vi "ListaStringParametros.vi"(2 "Tipo":T1, 4 "Parametros":variant) -> (16 "Parametros":string[](array[string]))   [LabVIEW 2017]
uses:
  Typedefs/Tipo_TipoSinalSimulado.ctl
  Typedefs/Tipo_ParamsRuido.ctl
  Typedefs/Tipo_ParamsFasor.ctl
  Typedefs/Tipo_ParamsSenoide.ctl
  Typedefs/Tipo_ParamsComposto.ctl
  Typedefs/Tipo_ComponenteSinalComposto.ctl
  Typedefs/Tipo_ParamsAMgen.ctl
  Typedefs/Tipo_ComponenteSinalRuidoComposto.ctl
  Typedefs/Tipo_TipoSinalCarrier.ctl
  Typedefs/Tipo_ParamsProximeter.ctl
  Typedefs/Tipo_ComponentesProximeter.ctl
  Typedefs/Tipo_ParamsEntreferro.ctl
  Typedefs/Tipo_ComponenteSinalEntreferro.ctl
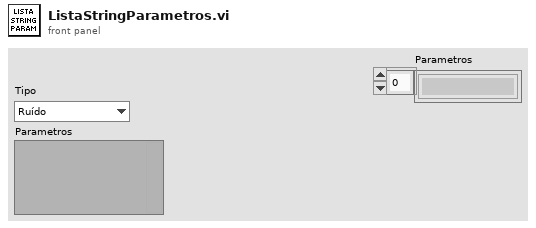
[diagram p1: front panel]
types:
  T1 = typedef "Tipo_TipoSinalSimulado.ctl" = enum16{"Ruído", "Fasor", "Senóide", "Composto", "AM", "Proximidade", "Entreferro"}
  T2 = typedef "Tipo_ParamsRuido.ctl" = cluster{"Amplitude":dbl, "Banda: ":bool, "Freq. Inferior":dbl, "Freq. Superior":dbl}
  T3 = typedef "Tipo_ParamsFasor.ctl" = cluster{"Amplitude Repouso":dbl, "Amplitude Pulso":dbl, "Freq. Pulsos":dbl, "Largura Pulsos":dbl}
  T4 = typedef "Tipo_ParamsSenoide.ctl" = cluster{"Amplitude":dbl, "Frequencia":dbl, "Fase":dbl}
  T5 = typedef "Tipo_ParamsComposto.ctl" = cluster{"Componentes":T6[], "Ruído":dbl}
  T6 = typedef "Tipo_ComponenteSinalComposto.ctl" = cluster{"Amplit.: ":dbl, "Freq. (Hz): ":dbl, "Fase (º):":dbl}
  T7 = typedef "Tipo_ParamsAMgen.ctl" = cluster{"Componentes":T8[], "Carrier Frequency":dbl, "Modulation":dbl, "Ruído Total":dbl, "Tipo":T9}
  T8 = typedef "Tipo_ComponenteSinalRuidoComposto.ctl" = cluster{"Amplit.: ":dbl, "Freq. (Hz): ":dbl, "Fase (º):":dbl, "Ruido":dbl}
  T9 = typedef "Tipo_TipoSinalCarrier.ctl" = enum16{"Ruído", "Senóide"}
  T10 = typedef "Tipo_ParamsProximeter.ctl" = cluster{"Rotacao":dbl, "Ruído":dbl, "Distância Eixo":dbl, "Fase":dbl, "Componentes":T11}
  T11 = typedef "Tipo_ComponentesProximeter.ctl" = cluster{"1xRPM":dbl, "2xRPM":dbl, "3xRPM":dbl, "4xRPM":dbl, "1/2xRPM":dbl, "1/3xRPM":dbl, "1/4xRPM":dbl, "0,45xRPM":dbl, "60Hz":dbl, "120Hz":dbl}
  T12 = typedef "Tipo_ParamsEntreferro.ctl" = cluster{"Componentes":T13[], "Num Polos":u16, "Folga Nominal":dbl, "Ruido":dbl, "Saturacao":dbl, "Angulo":dbl}
  T13 = typedef "Tipo_ComponenteSinalEntreferro.ctl" = cluster{"Pólo:":u16, "Amplitude:":dbl}
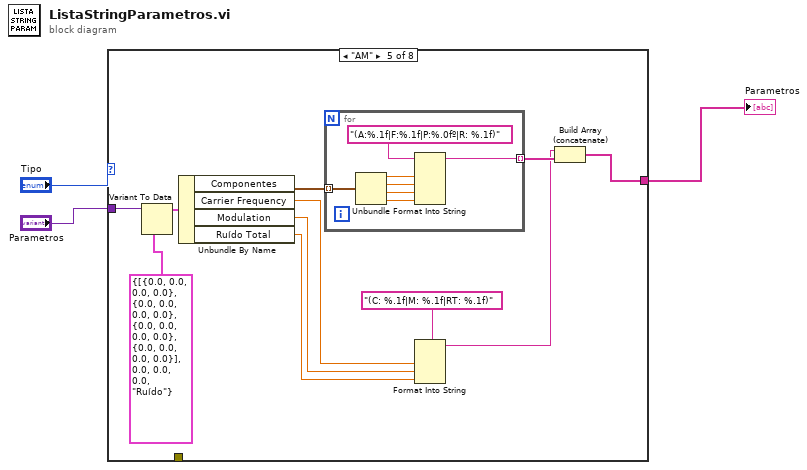
[diagram p0: block diagram]
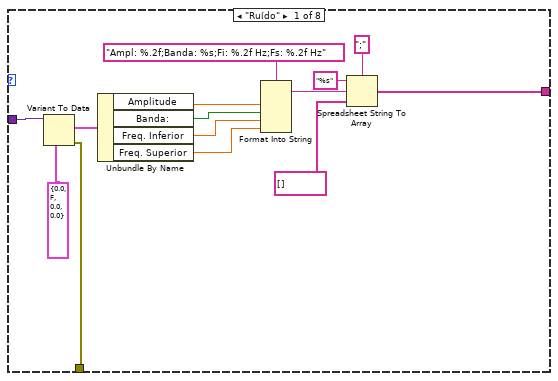
[diagram p2: hidden frame]
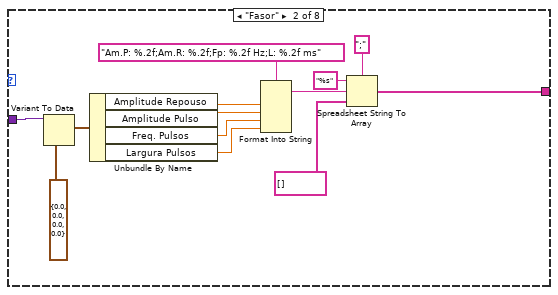
[diagram p3: hidden frame]
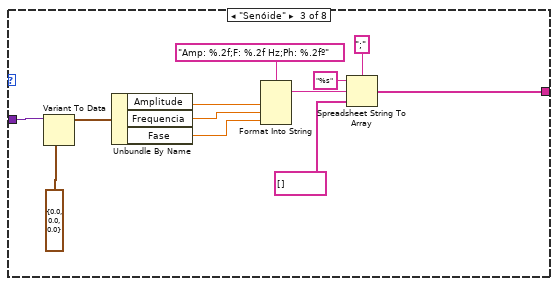
[diagram p4: hidden frame]
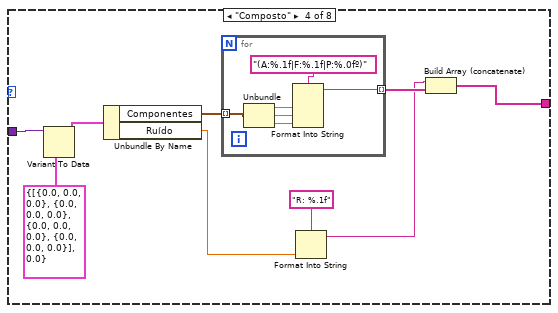
[diagram p5: hidden frame]
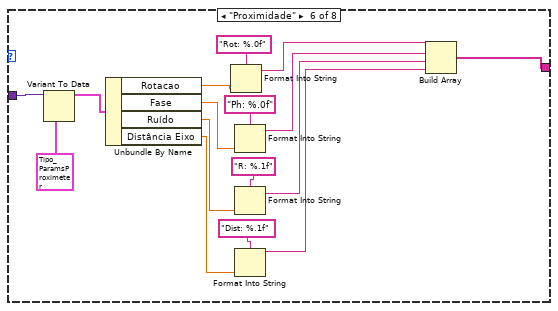
[diagram p6: hidden frame]
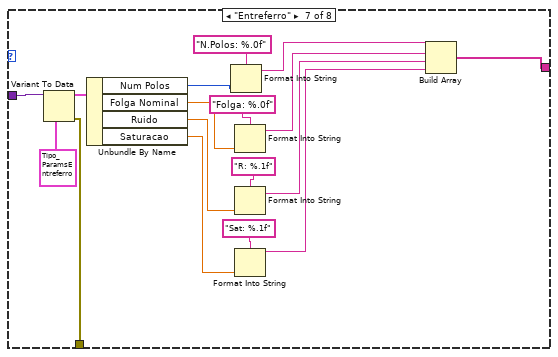
[diagram p7: hidden frame]
diagram:
  n1 = case shown="\"AM\"" "Tipo" {
    tunnel: "Parametros" -> [w17 w30 w42 w51 w64 w91 w108 _]
    tunnel: [w6 w19 w32 w46 w65 w76 w94 _] -> w1
    tunnel: [w4 _ _ _ _ _ w92 _] -> _
    frame "Ruído" {
      n2 = Variant To Data(type=T2 {"Amplitude"=0.0, "Banda: "=FALSE, "Freq. Inferior"=0.0, "Freq. Superior"=0.0} ("Tipo_ParamRuido"), Variant=w17) -> (data=w15:T2, error out=w4:errorcluster)  [unwired: 1 in]
      n3 = Unbundle By Name(w15) -> ("Amplitude"=w13:dbl, "Banda:"=w12:bool, "Freq. Inferior"=w11:dbl, "Freq. Superior"=w10:dbl)
      n4 = Format Into String(format string="Ampl: %.2f;Banda: %s;Fi: %.2f Hz;Fs: %.2f Hz", w13, w12, w11, w10) -> (resulting string=w9:string)  [unwired: 2 in, 1 out]
      n5 = Spreadsheet String To Array(delimiter (Tab)=";", format string="%s", spreadsheet string=w9, array type (2D Dbl)=string[] []) -> (array=w6:string[])
    }
    frame "Fasor" {
      n6 = Variant To Data(type=T3 {"Amplitude Repouso"=0.0, "Amplitude Pulso"=0.0, "Freq. Pulsos"=0.0, "Largura Pulsos"=0.0} ("Tipo_ParamRuido"), Variant=w30) -> (data=w28:T3)  [unwired: 1 in, 1 out]
      n7 = Unbundle By Name(w28) -> ("Amplitude Repouso"=w26:dbl, "Amplitude Pulso"=w25:dbl, "Freq. Pulsos"=w24:dbl, "Largura Pulsos"=w23:dbl)
      n8 = Format Into String(format string="Am.P: %.2f;Am.R: %.2f;Fp: %.2f Hz;L: %.2f ms", w26, w25, w24, w23) -> (resulting string=w22:string)  [unwired: 2 in, 1 out]
      n9 = Spreadsheet String To Array(delimiter (Tab)=";", format string="%s", spreadsheet string=w22, array type (2D Dbl)=string[] []) -> (array=w19:string[])
    }
    frame "Senóide" {
      n10 = Variant To Data(type=T4 {"Amplitude"=0.0, "Frequencia"=0.0, "Fase"=0.0} ("Tipo_ParamSenoide"), Variant=w42) -> (data=w40:T4)  [unwired: 1 in, 1 out]
      n11 = Unbundle By Name(w40) -> ("Amplitude"=w38:dbl, "Frequencia"=w37:dbl, "Fase"=w36:dbl)
      n12 = Format Into String(format string="Amp: %.2f;F: %.2f Hz;Ph: %.2fº", w38, w37, w36) -> (resulting string=w35:string)  [unwired: 2 in, 1 out]
      n13 = Spreadsheet String To Array(delimiter (Tab)=";", format string="%s", spreadsheet string=w35, array type (2D Dbl)=string[] []) -> (array=w32:string[])
    }
    frame "Composto" {
      n14 = Variant To Data(type=T5 {"Componentes"=[{"Amplit.: "=0.0, "Freq. (Hz): "=0.0, "Fase (º):"=0.0}, {"Amplit.: "=0.0, "Freq. (Hz): "=0.0, "Fase (º):"=0.0}, {"Amplit.: "=0.0, "Freq. (Hz): "=0.0, "Fase (º):"=0.0}, {"Amplit.: "=0.0, "Freq. (Hz): "=0.0, "Fase (º):"=0.0}], "Ruído"=0.0} ("Cluster"), Variant=w51) -> (data=w49:T5)  [unwired: 1 in, 1 out]
      n15 = Unbundle By Name(w49) -> ("Componentes"=w48:T6[], "Ruído"=w44:dbl)
      n16 = for {
        tunnel: w48 -> [w56] mode=indexing
        tunnel: [w52] -> w47 mode=indexing
        n17 = Unbundle(w56) -> ("Amplit.:"=w55:dbl, "Freq. (Hz):"=w54:dbl, "Fase (º):"=w53:dbl)
        n18 = Format Into String(format string="(A:%.1f|F:%.1f|P:%.0fº)", w55, w54, w53) -> (resulting string=w52:string)  [unwired: 2 in, 1 out]
      }
      n19 = Format Into String(format string="R: %.1f", w44) -> (resulting string=w43:string)  [unwired: 2 in, 1 out]
      n20 = Build Array (concatenate)(w43, w47) -> (w46:string[])
    }
    frame "AM" {
      n21 = Variant To Data(type=T7 {"Componentes"=[{"Amplit.: "=0.0, "Freq. (Hz): "=0.0, "Fase (º):"=0.0, "Ruido"=0.0}, {"Amplit.: "=0.0, "Freq. (Hz): "=0.0, "Fase (º):"=0.0, "Ruido"=0.0}, {"Amplit.: "=0.0, "Freq. (Hz): "=0.0, "Fase (º):"=0.0, "Ruido"=0.0}, {"Amplit.: "=0.0, "Freq. (Hz): "=0.0, "Fase (º):"=0.0, "Ruido"=0.0}], "Carrier Frequency"=0.0, "Modulation"=0.0, "Ruído Total"=0.0, "Tipo"=enum."Ruído"} ("Cluster"), Variant=w64) -> (data=w68:T7)  [unwired: 1 in, 1 out]
      n22 = Unbundle By Name(w68) -> ("Componentes"=w67:T8[], "Carrier Frequency"=w61:dbl, "Modulation"=w60:dbl, "Ruído Total"=w59:dbl)
      n23 = for {
        tunnel: w67 -> [w74] mode=indexing
        tunnel: [w70] -> w66 mode=indexing
        n24 = Unbundle(w74) -> ("Amplit.:"=w73:dbl, "Freq. (Hz):"=w72:dbl, "Fase (º):"=w71:dbl, "Ruido"=w69:dbl)
        n25 = Format Into String(format string="(A:%.1f|F:%.1f|P:%.0fº|R: %.1f)", w73, w72, w71, w69) -> (resulting string=w70:string)  [unwired: 2 in, 1 out]
      }
      n26 = Format Into String(initial string="(C: %.1f|M: %.1f|RT: %.1f)" ("format string"), w61, w60, w59) -> (resulting string=w58:string)  [unwired: 2 in, 1 out]
      n27 = Build Array (concatenate)(w58, w66) -> (w65:string[])
    }
    frame "Proximidade" {
      n28 = Variant To Data(type=T10 {"Rotacao"=0.0, "Ruído"=0.0, "Distância Eixo"=0.0, "Fase"=0.0, "Componentes"={"1xRPM"=0.0, "2xRPM"=0.0, "3xRPM"=0.0, "4xRPM"=0.0, "1/2xRPM"=0.0, "1/3xRPM"=0.0, "1/4xRPM"=0.0, "0,45xRPM"=0.0, "60Hz"=0.0, "120Hz"=0.0}} ("Tipo_ParamsProximeter"), Variant=w91) -> (data=w89:T10)  [unwired: 1 in, 1 out]
      n29 = Unbundle By Name(w89) -> ("Rotacao"=w87:dbl, "Fase"=w85:dbl, "Ruído"=w81:dbl, "Distância Eixo"=w79:dbl)
      n30 = Format Into String(format string="Rot: %.0f", w87) -> (resulting string=w84:string)  [unwired: 2 in, 1 out]
      n31 = Format Into String(format string="Ph: %.0f", w85) -> (resulting string=w83:string)  [unwired: 2 in, 1 out]
      n32 = Format Into String(format string="R: %.1f", w81) -> (resulting string=w78:string)  [unwired: 2 in, 1 out]
      n33 = Format Into String(format string="Dist: %.1f", w79) -> (resulting string=w77:string)  [unwired: 2 in, 1 out]
      n34 = Build Array(w84, w83, w78, w77) -> (w76:string[])
    }
    frame "Entreferro" {
      n35 = Variant To Data(type=T12 {"Componentes"=[{"Pólo:"=0, "Amplitude:"=0.0}, {"Pólo:"=0, "Amplitude:"=0.0}, {"Pólo:"=0, "Amplitude:"=0.0}, {"Pólo:"=0, "Amplitude:"=0.0}], "Num Polos"=0, "Folga Nominal"=0.0, "Ruido"=0.0, "Saturacao"=0.0, "Angulo"=0.0} ("Cluster"), Variant=w108) -> (data=w107:T12, error out=w92:errorcluster)  [unwired: 1 in]
      n36 = Unbundle By Name(w107) -> ("Num Polos"=w105:u16, "Folga Nominal"=w103:dbl, "Ruido"=w99:dbl, "Saturacao"=w97:dbl)
      n37 = Format Into String(format string="N.Polos: %.0f", w105) -> (resulting string=w102:string)  [unwired: 2 in, 1 out]
      n38 = Format Into String(format string="Folga: %.0f", w103) -> (resulting string=w101:string)  [unwired: 2 in, 1 out]
      n39 = Format Into String(format string="R: %.1f", w99) -> (resulting string=w96:string)  [unwired: 2 in, 1 out]
      n40 = Format Into String(format string="Sat: %.1f", w97) -> (resulting string=w95:string)  [unwired: 2 in, 1 out]
      n41 = Build Array(w102, w101, w96, w95) -> (w94:string[])
    }
    frame Default {
    }
  }
  "Parametros" <- w1
